vi "Stop Core.vi"(10 "final error code":i32, 11 "Cobra RT in":refnum<class "Cobra RT.lvclass">) -> (3 "Cobra RT out":refnum<class "Cobra RT.lvclass">)   [LabVIEW 2019, in "Cobra RT.lvlib" / "Cobra RT.lvclass"]
doc: "(<B>Filename</B>: Actor Framework.lvlib:Actor.lvclass:Stop Core.vi)\n\nDefines what the actor does before it stops. Use the <B>final error code</B> input to determine whether the actor shut down in response to an error.\n\nBy default, this method passes the Stop message along to all auto-stop nested actors. A descendant class may override this method to define additional behavior, such as shutting down any processes the actor initiated in its override of the Actor Core method."
uses:
  Cobra RT.lvclass
  Cobra RT.lvclass/Cobra RT.ctl
  <vilib>/MGI/Panel Manager/Panel Actor/Panel Actor/Panel Actor.lvclass
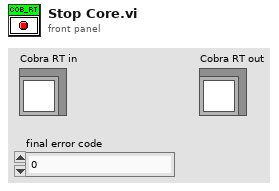
[diagram p1: front panel]
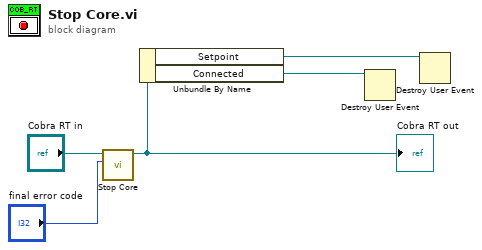
[diagram p0: block diagram]
diagram:
  n1 = call-parent "Stop Core.vi"("final error code"="final error code", "Monitored Actor in"="Cobra RT in") -> ("Monitored Actor out"=w3:refnum<class "Cobra RT.lvclass">)  [unwired: 9 in]
  "Cobra RT out" <- w3
  n2 = Unbundle By Name(w3) -> ("Setpoint"=w1:refnum<user-event>, "Connected"=w2:refnum<user-event>)
  n3 = Destroy User Event(user event=w2) -> ()  [unwired: 1 in, 1 out]
  n4 = Destroy User Event(user event=w1) -> ()  [unwired: 1 in, 1 out]
